vi "get_web_events.vi"(8 "error in (no error)":errorcluster, 11 "simple_html_chat_ui in":refnum<class "simple_html_chat_ui.lvclass">) -> (0 "error out":errorcluster, 2 "Web Events":T1, 3 "simple_html_chat_ui out":refnum<class "simple_html_chat_ui.lvclass">)   [LabVIEW 2020, in "simple_html_chat_ui.lvclass"]
uses:
  simple_html_chat_ui.lvclass
  typedefs/web_events.ctl
  models/abstract_message_base/abstract_message_base.lvclass
  simple_html_chat_ui.lvclass/simple_html_chat_ui.ctl
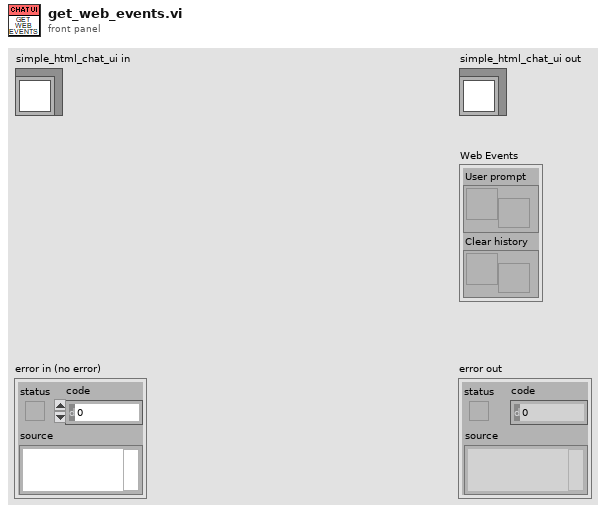
[diagram p1: front panel]
types:
  T1 = typedef "simple_html_chat_ui.lvclass/web_events.ctl" = cluster{"User prompt":refnum<user-event>, "Clear history":refnum<user-event>}
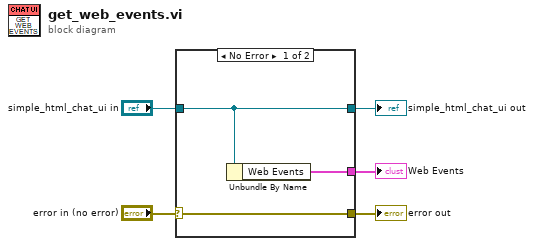
[diagram p0: block diagram]
diagram:
  n1 = case shown="No Error" "error in (no error)" {
    selector: "error in (no error)" -> [w8 w10]
    tunnel: [w8 w10] -> w4
    tunnel: [w7 w9] -> w2
    tunnel: "simple_html_chat_ui in" -> [w7 w9]
    tunnel: [w6 _] -> w1
    frame No Error {
      n2 = Unbundle By Name(w7) -> ("Web Events"=w6:T1)
    }
    frame Error {
    }
  }
  "error out" <- w4
  "simple_html_chat_ui out" <- w2
  "Web Events" <- w1
